vi "Task ID.vi"(8 "error in (no error)":errorcluster, 11 "DataHandlerTask in":refnum<class "DataHandlerTask.lvclass">) -> (0 "error out":errorcluster, 2 "Task ID":string, 3 "DataHandlerTask out":refnum<class "DataHandlerTask.lvclass">)   [LabVIEW 2020, in "VolatusData.lvlib" / "DataHandlerTask.lvclass"]
uses:
  DataHandlerTask.lvclass
  DataHandlerTask.lvclass/DataHandlerTask.ctl
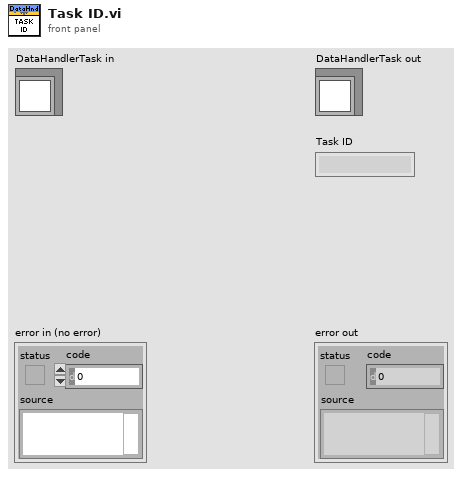
[diagram p1: front panel]
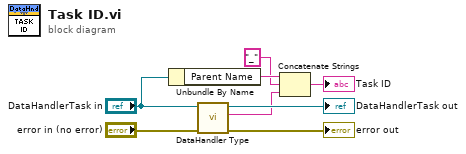
[diagram p0: block diagram]
diagram:
  n1 = Unbundle By Name("DataHandlerTask in") -> ("Parent Name"=w4:string)
  n2 = call-dynamic "DataHandler Type.vi"("error in (no error)"="error in (no error)", "DataHandlerTask in"="DataHandlerTask in") -> ("error out"=→"error out":errorcluster, "DataHandler Type"=w2:string, "DataHandlerTask out"=→"DataHandlerTask out":refnum<class "DataHandlerTask.lvclass">)  [unwired: 7 in]
  n3 = Concatenate Strings(w4, "_" ("string"), w2) -> (→"Task ID":string)
